vi "ziusb.vi"() -> ()   [LabVIEW 2016]
panel:
  out "读取缓冲区 2":string
  in  "写入缓冲区 2":string
  out "读取缓冲区":string
  in  "写入缓冲区":string
  in  "布尔":bool
  in  "VISA资源名称 2":refnum<visa-resource-name>
  in  "VISA资源名称":refnum<visa-resource-name>
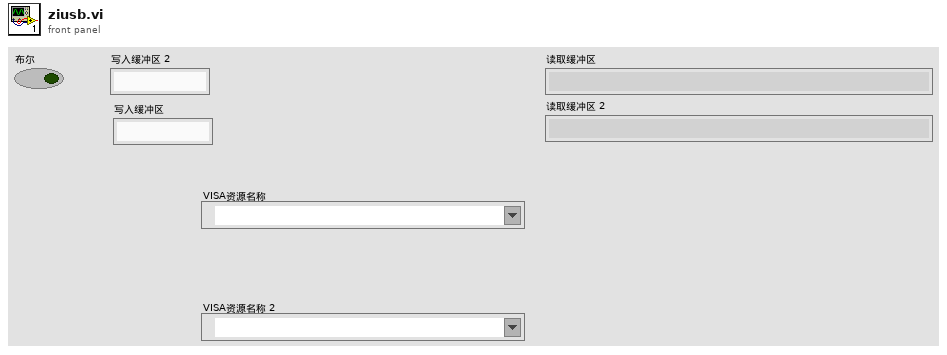
[diagram p1: front panel]
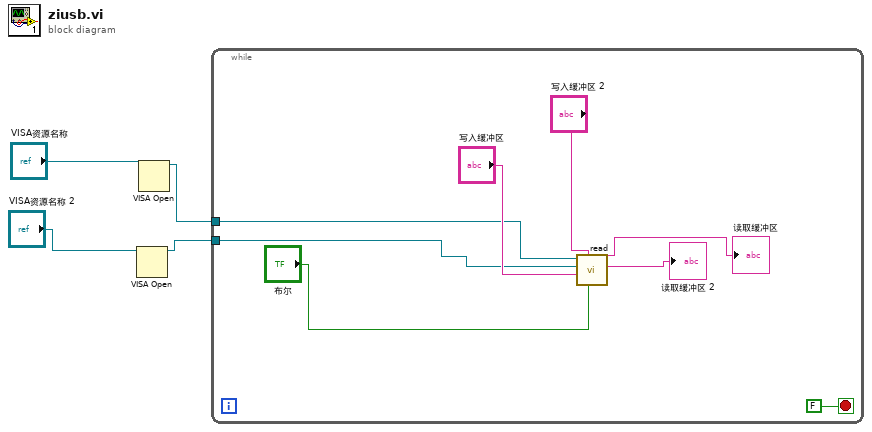
[diagram p0: block diagram]
diagram:
  n1 = VISA Open(VISA resource name="VISA资源名称 2") -> (VISA resource name=w1:refnum<visa-resource-name>)  [unwired: 4 in, 1 out]
  n2 = VISA Open(VISA resource name="VISA资源名称") -> (VISA resource name=w2:refnum<visa-resource-name>)  [unwired: 4 in, 1 out]
  n3 = while {
    tunnel: w2 -> [w6]
    tunnel: w1 -> [w5]
    stop <- FALSE stop-if-true
    n4 = call "read.vi"("布尔"="布尔", "写入缓冲区 2"="写入缓冲区 2", "写入缓冲区"="写入缓冲区", "VISA资源名称输入"=w5, "VISA引用句柄输入"=w6) -> ("读取缓冲区 2"=→"读取缓冲区 2":string, "读取缓冲区"=→"读取缓冲区":string)  [unwired: 5 in]
  }
